vi "niRFUtil WFM Align Waveforms - Coarse (real wfm).vi"(0 "Waveform In":T1 {"y" min=0 max=127 format="%.2f"; "dx" format="%^.2e"; "x0" format="%^.2e"}, 5 "Reference Waveform":T1 {"y" min=0 max=127 format="%.2f"; "dx" format="%^.2e"; "x0" format="%^.2e"}, 7 "Window Start, sec":dbl format="%^.2e", 9 "Window Duration, sec":dbl format="%^.2e") -> (4 "Waveform Out":T1 {"y" min=0 max=127 format="%.2f"; "dx" format="%^.2e"; "x0" format="%^.2e"})   [LabVIEW 2015, in "niRFUtil.lvlib"]
doc: "(c) Copyright 2006, National Instruments, Inc. This VI may not be duplicated, sold, or distributed without written consent from National Instruments."
uses:
  niRFUtil.lvlib
  Includes/niRFUtil INC Real Waveform.ctl
  Includes/niRFUtil INC Real Array.ctl
  niRFUtil WFM Parse Waveform - Duration (real wfm).vi
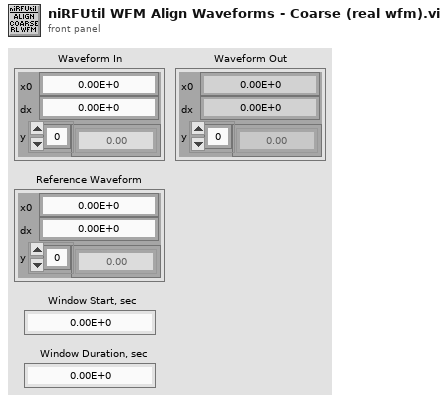
[diagram p1: front panel]
types:
  T1 = typedef "niRFUtil.lvlib/niRFUtil INC Real Waveform.ctl" = cluster{"x0":dbl, "dx":dbl, "y":T2}
  T2 = typedef "niRFUtil.lvlib/niRFUtil INC Real Array.ctl" = sgl[]
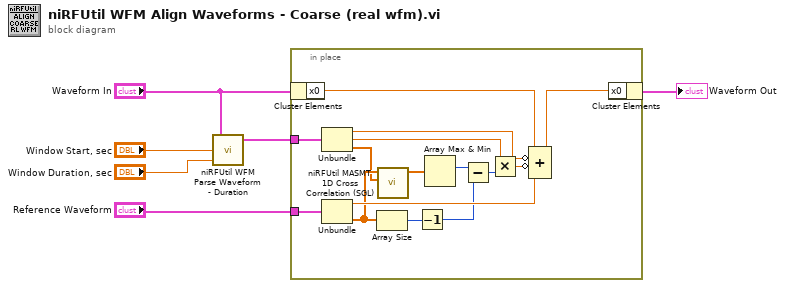
[diagram p0: block diagram]
diagram:
  n1 = call-poly "niRFUtil WFM Parse Waveform - Duration.vi"("Duration (Inf)"="Window Duration, sec", "Start (-Inf)"="Window Start, sec", "Waveform In"="Waveform In") -> ("Waveform Out"=w3:T1)  [unwired: 2 out]
  n2 = in-place {
    in-place-border: "Reference Waveform" -> [w21]
    in-place-border: w3 -> [w20]
    n3 = in-place-cluster #1("Waveform In") -> ("x0"=w8:dbl)
    n4 = Unbundle(w20) -> ("x0"=w13:dbl, "dx"=w17:dbl, "y"=w10:T2)
    n5 = Unbundle(w21) -> ("x0"=w15:dbl, "y"=w11:T2)  [unwired: 1 out]
    n6 = Array Size(array=w11) -> (size(s)=w14:i32)
    n7 = call "niRFUtil MASMT 1D Cross Correlation (SGL).vi"("Y"=w10, "X"=w11) -> ("Rxy"=w9:sgl[])  [unwired: 8 in, 1 out]
    n8 = Decrement(x=w14) -> (x-1=w12:i32)
    n9 = Array Max & Min(array=w9) -> (max index (indices)=w19:i32)  [unwired: 3 out]
    n10 = Subtract(x=w19, y=w12) -> (x-y=w18:i32)
    n11 = Multiply(x=w17, y=w18) -> (x*y=w16:dbl)
    n12 = Compound Arithmetic op=ADD(w8, invert w13, invert w16, w15) -> (w7:dbl)
    n13 = in-place-cluster #1("x0"=w7) -> (→"Waveform Out":T1)
  }
